vi "Tell Stopped.vi"(8 "Error in":errorcluster, 10 "Actor":refnum<class "Actor.lvclass">) -> ()   [LabVIEW 2025, in "jettl.lvlib" / "Actor.lvlib"]
uses:
  Actor.lvlib
  Actor/Actor.lvclass
  Stopped Msg/Tell Parent.vi
  Stopped Msg/Tell Child.vi
  Stopped Msg/Stopped Msg.lvlib
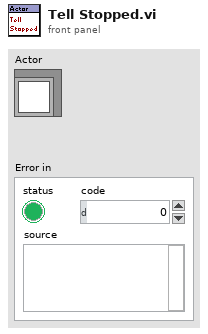
[diagram p1: front panel]
types:
  T1 = typedef "jettl.lvlib/Actor.lvlib/Child UIDs.ctl" = set{string}
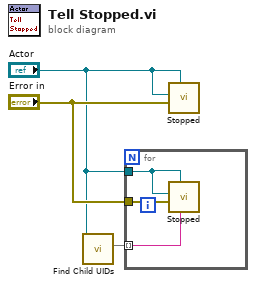
[diagram p0: block diagram]
diagram:
  n1 = call-dynamic "Find Child UIDs.vi"("Actor in"="Actor") -> ("Child UIDs"=w3:T1)  [unwired: 10 in]
  n2 = for {
    tunnel: "Actor" -> [w6]
    tunnel: w3 -> [w4] mode=indexing
    tunnel: "Error in" -> [w5]
    n3 = call-poly "Stopped.vi"("UID"=w4, "Actor in"=w6, "Error"=w5, "Actor"=w6) -> ()  [unwired: 7 in, 1 out]
  }
  n4 = call-poly "Stopped.vi"("Actor in"="Actor", "Error"="Error in", "Actor"="Actor") -> ()  [unwired: 8 in, 1 out]
